vi "Read channel pattern matches.vi"(8 "error in (no error)":errorcluster, 11 "TDMS datalogger configuration in":refnum<class "TDMS datalogger configuration.lvclass">) -> (0 "error out":errorcluster, 2 "channel pattern matches":string[](array[string]), 3 "TDMS datalogger configuration out":refnum<class "TDMS datalogger configuration.lvclass">)   [LabVIEW 2015, in "TDMS datalogger configuration.lvclass"]
uses:
  TDMS datalogger configuration.lvclass
  TDMS datalogger configuration.lvclass/TDMS datalogger configuration.ctl
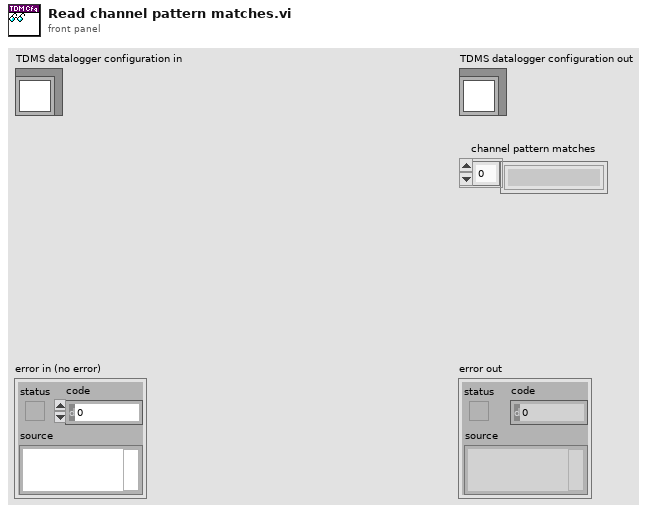
[diagram p1: front panel]
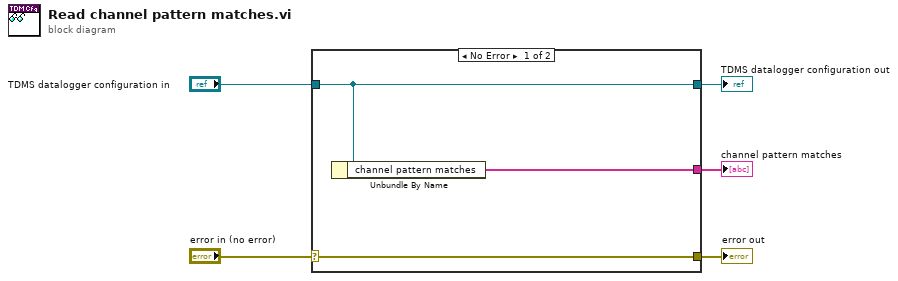
[diagram p0: block diagram]
diagram:
  n1 = case shown="No Error" "error in (no error)" {
    selector: "error in (no error)" -> [w8 w9]
    tunnel: [w8 w9] -> w4
    tunnel: [w7 w10] -> w2
    tunnel: "TDMS datalogger configuration in" -> [w7 w10]
    tunnel: [w6 _] -> w1
    frame No Error {
      n2 = Unbundle By Name(w7) -> ("channel pattern matches"=w6:string[])
    }
    frame Error {
    }
  }
  "error out" <- w4
  "TDMS datalogger configuration out" <- w2
  "channel pattern matches" <- w1
